vi "UpdateStatusLog.vi"(8 "error in (no error)":errorcluster, 10 "Data":string, 11 "CameraTestingUI in":refnum<class "CameraTestingUI.lvclass">) -> (0 "error out":errorcluster, 3 "CameraTestingUI out":refnum<class "CameraTestingUI.lvclass">)   [LabVIEW 2020, in "CameraTestingUI.lvlib" / "CameraTestingUI.lvclass"]
uses:
  CameraTestingUI.lvclass
  CameraTestingUI.lvclass/CameraTestingUI.ctl
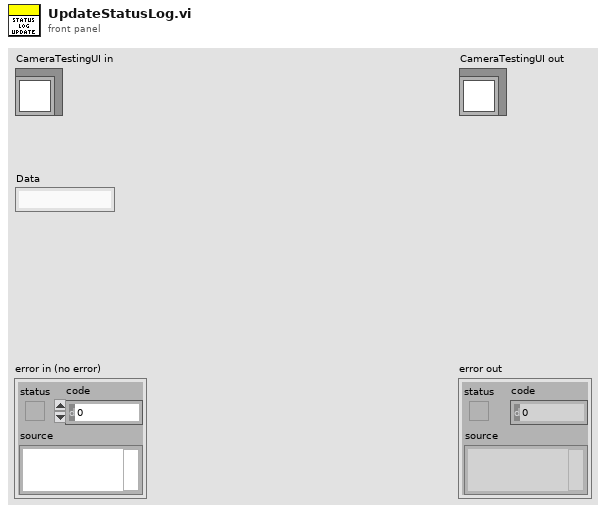
[diagram p1: front panel]
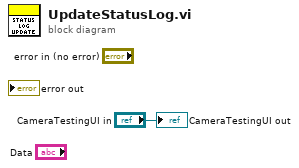
[diagram p0: block diagram]
diagram:
  "CameraTestingUI out" <- "CameraTestingUI in"
